vi "Initialize Attributes.vi"(8 "error in (no error)":errorcluster, 10 "Attribute Data":variant, 11 "CS++GoBangClient in":refnum<class "CS++GoBangClient.lvclass">) -> (0 "error out":errorcluster, 2 "Found?":bool, 3 "CS++GoBangClient out":refnum<class "CS++GoBangClient.lvclass">)   [LabVIEW 2014, in "GoBang.lvlib" / "CS++GoBangClient.lvclass"]
doc: "Initialize object attribute.\n\nUnique resources should be allocated elsewhere!"
uses:
  CS++GoBangClient.lvclass
  CS++GoBangClient.lvclass/CS++GoBangClient.ctl
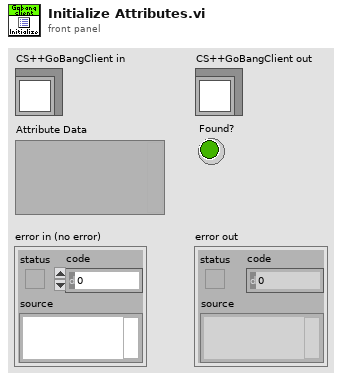
[diagram p1: front panel]
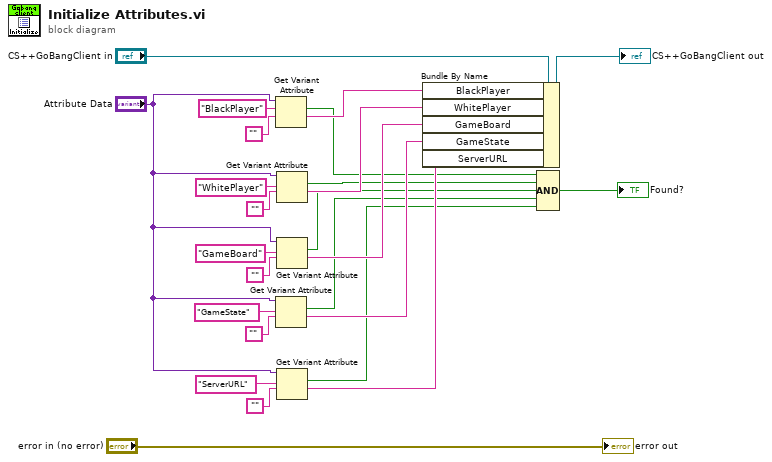
[diagram p0: block diagram]
diagram:
  n1 = Get Variant Attribute(Variant="Attribute Data", name="BlackPlayer", default value (empty Variant)="") -> (found=w7:bool, value=w15:string)  [unwired: 1 in, 2 out]
  n2 = Get Variant Attribute(Variant="Attribute Data", name="GameState", default value (empty Variant)="") -> (found=w4:bool, value=w12:string)  [unwired: 1 in, 2 out]
  n3 = Get Variant Attribute(Variant="Attribute Data", name="WhitePlayer", default value (empty Variant)="") -> (found=w6:bool, value=w14:string)  [unwired: 1 in, 2 out]
  n4 = Get Variant Attribute(Variant="Attribute Data", name="GameBoard", default value (empty Variant)="") -> (found=w5:bool, value=w13:string)  [unwired: 1 in, 2 out]
  n5 = Get Variant Attribute(Variant="Attribute Data", name="ServerURL", default value (empty Variant)="") -> (found=w3:bool, value=w8:string)  [unwired: 1 in, 2 out]
  n6 = Bundle By Name(cluster="CS++GoBangClient in", "BlackPlayer"=w15, "WhitePlayer"=w14, "GameBoard"=w13, "GameState"=w12, "ServerURL"=w8) -> (→"CS++GoBangClient out":refnum<class "CS++GoBangClient.lvclass">)
  n7 = Compound Arithmetic op=AND(w7, w6, w5, w4, w3) -> (→"Found?":bool)
  "error out" <- "error in (no error)"
